vi "createQuery.vi"(8 "error in (no error)":errorcluster, 10 "queries":T1, 11 "DomeCommunicator in":refnum<class "DomeCommunicator.lvclass">) -> (0 "error out":errorcluster, 2 "query":string, 3 "DomeCommunicator out":refnum<class "DomeCommunicator.lvclass">)   [LabVIEW 2016, in "DomeCommunicator.lvclass"]
uses:
  DomeCommunicator.lvclass
  ComTypedefs/queries.ctl
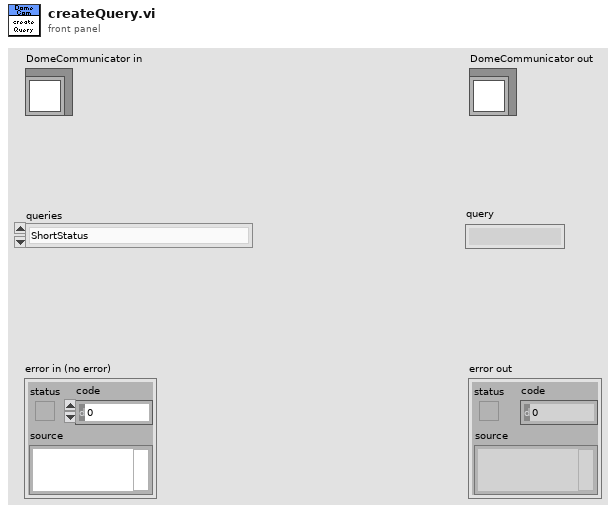
[diagram p1: front panel]
types:
  T1 = typedef "queries.ctl" = enum16{"ShortStatus", "FullEngineeringStatus", "RecallLastSavedConfiguration"}
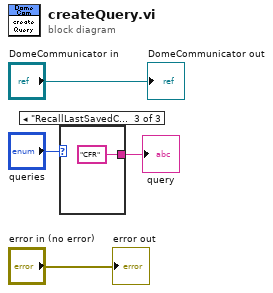
[diagram p0: block diagram]
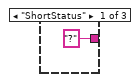
[diagram p2: hidden frame]
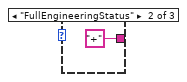
[diagram p3: hidden frame]
diagram:
  n1 = case shown="\"RecallLastSavedConfiguration\"" "queries" {
    tunnel: ["?" ("query") "+" ("query") "CFR" ("query")] -> w1
    frame "ShortStatus" {
    }
    frame "FullEngineeringStatus" {
    }
    frame "RecallLastSavedConfiguration" {
    }
  }
  "query" <- w1
  "error out" <- "error in (no error)"
  "DomeCommunicator out" <- "DomeCommunicator in"
